vi "Stop Core.vi"(10 "final error code":i32, 11 "Island Watch in":refnum<class "Island Watch.lvclass">) -> (3 "Island Watch out":refnum<class "Island Watch.lvclass">)   [LabVIEW 2015, in "Island Watch Actor.lvlib" / "Island Watch.lvclass"]
doc: "(<B>Filename</B>: Actor Framework.lvlib:Actor.lvclass:Stop Core.vi)\n\nDefines what the actor does before it stops. Use the <B>final error code</B> input to determine whether the actor shut down in response to an error.\n\nBy default, this method does nothing. A descendant class may override it to define behavior, such as shutting down any processes the actor initiated in its override of the Actor Core method."
uses:
  Island Watch.lvclass
  Island Watch.lvclass/Island Watch.ctl
  <vilib>/ActorFramework/Actor/Actor.lvclass
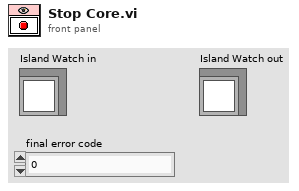
[diagram p1: front panel]
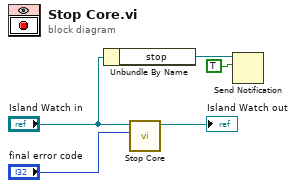
[diagram p0: block diagram]
diagram:
  n1 = Unbundle By Name("Island Watch in") -> ("stop"=w2:refnum<notifier>)
  n2 = call-parent "Stop Core.vi"("final error code"="final error code", "Actor in"="Island Watch in") -> ("Actor out"=→"Island Watch out":refnum<class "Island Watch.lvclass">)  [unwired: 9 in]
  n3 = Send Notification(notification=TRUE, notifier=w2) -> ()  [unwired: 1 in, 2 out]
